vi "Create-Order.vi"(11 "Command":T1={"Side"=enum."Sell", "Operation"=enum."AddOrder", "Price"=139.42, "# of Shares"=300, "OrderRefNum"=12379813738319119367}) -> (3 "Array":u64[](array[numeric]) format="%.0x")   [LabVIEW 2016]
uses:
  Host-Command-for-Fpga.ctl
panel:
  out "Price":u32 format="%.0x"
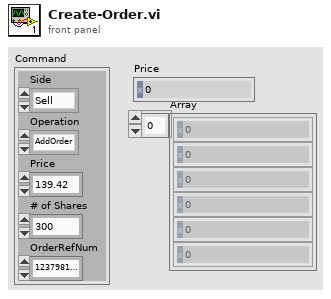
[diagram p1: front panel]
types:
  T1 = typedef "Host-Command-for-Fpga.ctl" = cluster{"Side":enum16{"Buy", "Sell"}, "Operation":enum16{"GetAll", "AddOrder", "DeleteOrder"}, "Price":dbl, "# of Shares":u32, "OrderRefNum":u64}
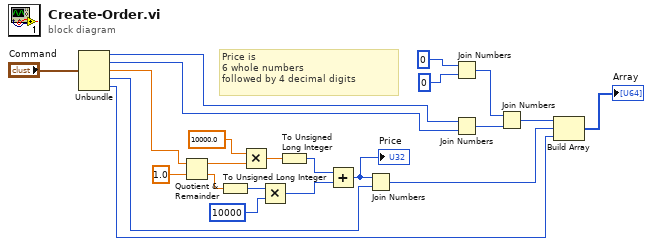
[diagram p0: block diagram]
diagram:
  # "Price is\n6 whole numbers\nfollowed by 4 decimal digits"
  n1 = Unbundle("Command") -> ("Side"=w1:enum16{"Buy", "Sell"}, "Operation"=w5:enum16{"GetAll", "AddOrder", "DeleteOrder"}, "Price"=w4:dbl, "# of Shares"=w3:u32, "OrderRefNum"=w2:u64)
  n2 = Quotient & Remainder(x=w4, y=1.0) -> (x-y*floor(x/y)=w14:dbl, floor(x/y)=w15:dbl)
  n3 = To Unsigned Long Integer(number=w15) -> (unsigned 32bit integer=w20:u32)
  n4 = Multiply(x=10000.0, y=w14) -> (x*y=w16:dbl)
  n5 = Multiply(x=w20, y=u32 10000 ("x")) -> (x*y=w19:u32)
  n6 = To Unsigned Long Integer(number=w16) -> (unsigned 32bit integer=w18:u32)
  n7 = Add(x=w18, y=w19) -> (x+y=w22:u32)
  "Price" <- w22
  n8 = Join Numbers(hi=w22, lo=w3) -> ((hi.lo)=w23:u64)
  n9 = Join Numbers(hi=u16 0, lo=u16 0) -> ((hi.lo)=w10:u32)
  n10 = Join Numbers(hi=w1, lo=w5) -> ((hi.lo)=w8:u32)
  n11 = Join Numbers(hi=w10, lo=w8) -> ((hi.lo)=w9:u64)
  n12 = Build Array(w9, w23, w2) -> (→"Array":u64[])
